vi "Probe-Variant As Tree.vi"(11 "VAttributes":variant) -> (2 "Value String":string, 3 "Boolean":bool)   [LabVIEW 2019]
uses:
  lv-apt-json-file.lvlib
panel:
  in  "Tree":string(tree)
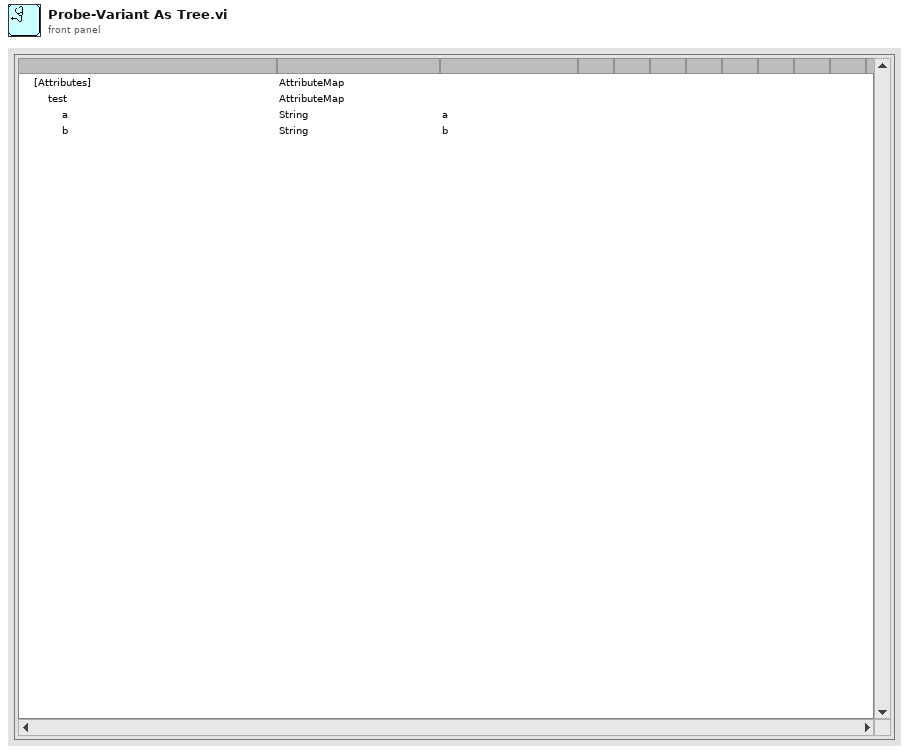
[diagram p1: front panel]
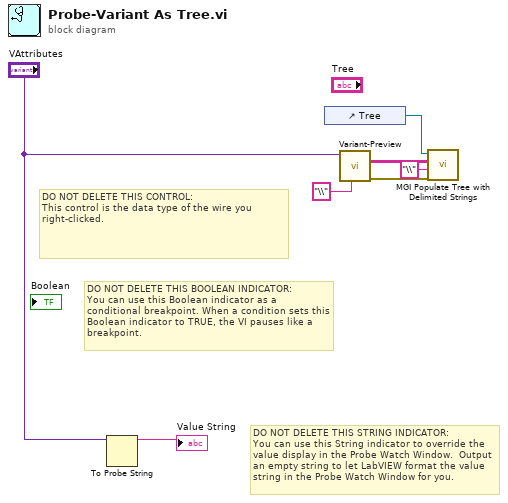
[diagram p0: block diagram]
diagram:
  # "DO NOT DELETE THIS STRING INDICATOR: \nYou can use this String indicator to override the value display in the Probe Watch Window.  Output an empty string to let LabVIEW format the value string in the Probe Watch Window for you."
  # "DO NOT DELETE THIS BOOLEAN INDICATOR: \nYou can use this Boolean indicator as a conditional breakpoint. When a condition sets this Boolean indicator to TRUE, the VI pauses like a breakpoint."
  # "DO NOT DELETE THIS CONTROL: \nThis control is the data type of the wire you right-clicked."
  n1 = To Probe String(7:"VAttributes") -> (3:→"Value String":string)  [unwired: 2 in, 1 out]
  n2 = control-ref of="Tree"() -> (w5:refnum<vi>)
  n3 = call "Variant-Preview.vi"("delimiter (/)"="\\", "data"="VAttributes") -> ("error out"=w6:errorcluster, "Array"=w4:string[][])  [unwired: 7 in, 1 out]
  n4 = call <userlib>:"MGI Populate Tree with Delimited Strings.vi"("error in (no error)"=w6, "Delimiter"="\\", "Items (Delimited)"=w4, "Tree Control"=w5) -> ()  [unwired: 5 in, 3 out]
